vi "Error_csv_to_ram.vi"(6 "pattern":string="error*-*.csv", 8 "error in (no error)":errorcluster, 11 "file path (use dialog)":path) -> (0 "error out":errorcluster, 3 "array":string[][](array[string]))   [LabVIEW 2012]
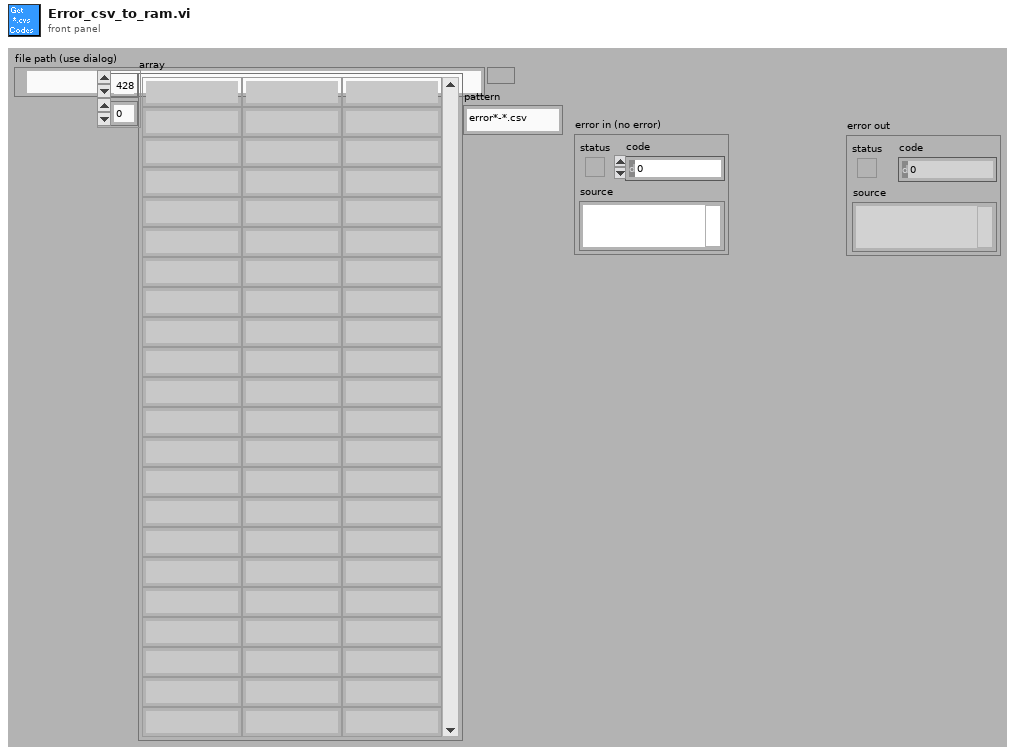
[diagram p1: front panel]
types:
  T1 = enum16{"open", "replace", "create", "open or create", "replace or create", "replace or create with confirmation"}
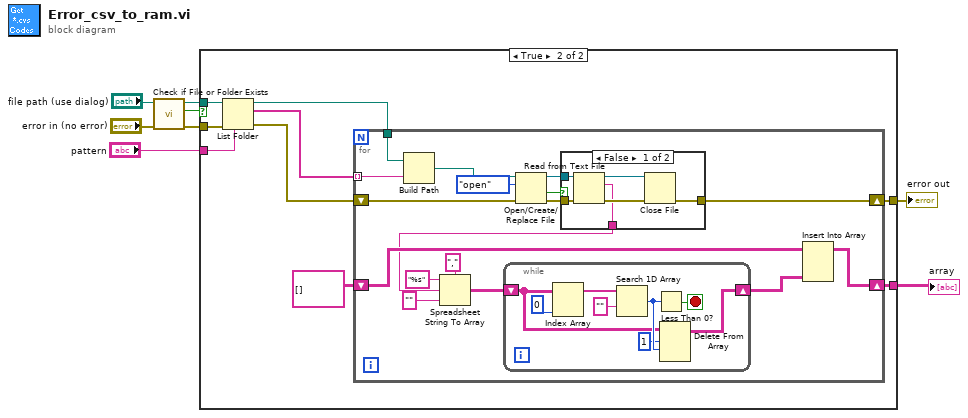
[diagram p0: block diagram]
diagram:
  n1 = call <vilib>:"Check if File or Folder Exists.vi"("error in (no error)"="error in (no error)", "path"="file path (use dialog)") -> ("error out"=w4:errorcluster, "file or folder exists?"=w1:bool, "dup path"=w3:path)  [unwired: 7 in]
  n2 = case shown="True" w1 {
    tunnel: "pattern" -> [_ w18]
    tunnel: [_ w14] -> w7
    tunnel: [w9 w12] -> w6
    tunnel: w4 -> [w9 w11]
    tunnel: w3 -> [_ w10]
    frame False {
    }
    frame True {
      n3 = List Folder(path=w10, pattern=w18, error in=w11) -> (path out=w15:path, filenames=w16:string[], error out=w17:errorcluster)  [unwired: 1 in, 1 out]
      n4 = for {
        tunnel: w16 -> [w32] mode=indexing
        shift-right: [w27] -> w12
        shift-left: w17 -> [w28]
        tunnel: w15 -> [w25]
        shift-right: [w23] -> w14
        shift-left: string[][] [] -> [w24]
        n5 = Build Path(base path=w25, name or relative path=w32) -> (appended path=w26:path)
        n6 = Open/Create/Replace File(file path (use dialog)=w26, error in=w28, operation (0:open)=T1."open") -> (refnum out=w31:refnum<file>, cancelled=w19:bool, error out=w29:errorcluster)  [unwired: 3 in]
        n7 = case shown="False" w19 {
          tunnel: w31 -> [w41 _]
          tunnel: w29 -> [w40 w42]
          tunnel: [w37 w42] -> w27
          tunnel: [w36 _] -> w22
          frame False {
            n8 = Read from Text File(file (use dialog)=w41, error in=w40) -> (refnum out=w39:refnum<file>, text=w36:string, error out=w38:errorcluster)  [unwired: 2 in, 1 out]
            n9 = Close File(refnum=w39, error in=w38) -> (error out=w37:errorcluster)  [unwired: 1 out]
          }
          frame True {
          }
        }
        n10 = Spreadsheet String To Array(delimiter (Tab)=",", format string="%s", spreadsheet string=w22, array type (2D Dbl)="") -> (array=w21:string[][])
        n11 = while {
          shift-right: [w44] -> w20
          shift-left: w21 -> [w46]
          stop <- w49 stop-if-true
          n12 = Index Array(array=w46, index (col)=0 ("index (row)")) -> (element=w45:string[])  [unwired: 1 in]
          n13 = Search 1D Array(1D array=w45, element="") -> (index of element=w48:i32)  [unwired: 1 in]
          n14 = Less Than 0?(x=w48) -> (x < 0?=w49:bool)
          n15 = Delete From Array(array=w46, length=1, index (row)=w48) -> (array with subset deleted=w44:string[][])  [unwired: 1 in, 1 out]
        }
        n16 = Insert Into Array(array=w24, new element=w20) -> (w23:string[][])  [unwired: 2 in]
      }
    }
  }
  "array" <- w7
  "error out" <- w6
